vi "createTuplaEnDBImage.vi"(0 "claseImagen in":refnum<class "claseImagen.lvclass">, 3 "error in":errorcluster) -> (7 "claseImagen out":refnum<class "claseImagen.lvclass">, 10 "error out":errorcluster)   [LabVIEW 2014, in "claseImagen.lvclass"]
uses:
  claseImagen.lvclass
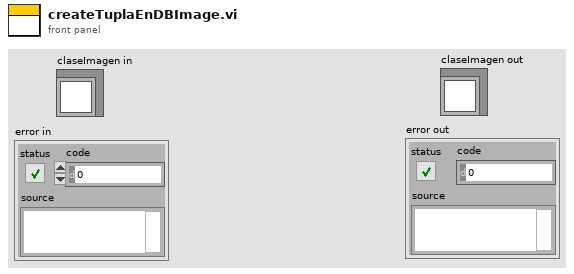
[diagram p1: front panel]
types:
  T1 = cluster{"idImage":dbl, "camposDeMedicionImage":string, "dateCreateImage":timestamp}
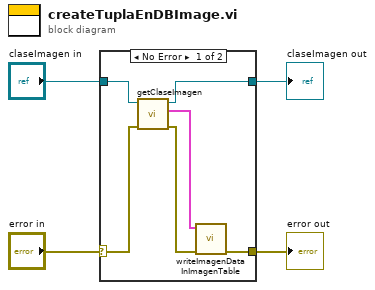
[diagram p0: block diagram]
diagram:
  n1 = case shown="No Error" "error in" {
    selector: "error in" -> [w9 w12]
    tunnel: [w6 w12] -> w3
    tunnel: [w5 w11] -> w2
    tunnel: "claseImagen in" -> [w10 w11]
    frame No Error {
      n2 = call "getClaseImagen.vi"("error in"=w9, "claseImagen in"=w10) -> ("error out"=w7:errorcluster, "dataReading"=w8:T1, "claseImagen out"=w5:refnum<class "claseImagen.lvclass">)  [unwired: 7 in]
      n3 = call "writeImagenDataInImagenTable.vi"("error in"=w7, "dataToWrite"=w8) -> ("error out"=w6:errorcluster)  [unwired: 9 in]
    }
    frame Error {
    }
  }
  "claseImagen out" <- w2
  "error out" <- w3
